vi "ideal_inverse_kinematics.vi"(11 "Pose":T1) -> (3 "Axis positions":dbl[](array[numeric]))   [LabVIEW 2011]
uses:
  <vilib>/Analysis/Matrix/Datatypes/RealMatrix.ctl
  <vilib>/Analysis/baseanly.llb/A x Vector.vi
  <vilib>/Analysis/NI_AALBase.lvlib
  <vilib>/Analysis/Matrix/NI_Matrix.lvlib
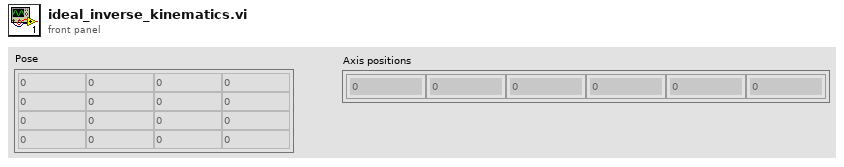
[diagram p1: front panel]
types:
  T1 = typedef "NI_Matrix.lvlib/RealMatrix.ctl" = dbl[][]
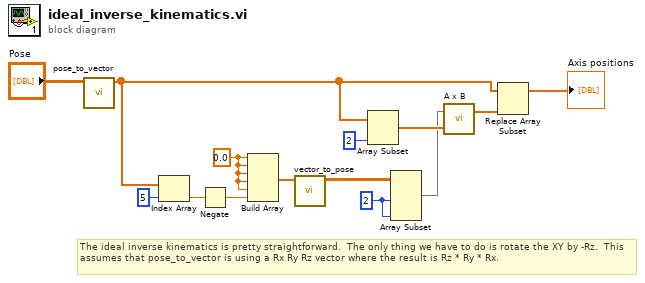
[diagram p0: block diagram]
diagram:
  w8 = 2 ("length")
  w3 = 0.0 ("element")
  # "The ideal inverse kinematics is pretty straightforward.  The only thing we have to do is rotate the XY by -Rz.  This assumes that pose_to_vector is using a Rx Ry Rz vector where the result is Rz * Ry * Rx."
  n1 = call "pose_to_vector.vi"("Pose"="Pose") -> ("Pose vector"=w13:dbl[])  [unwired: 10 in]
  n2 = Index Array(array=w13, index=5) -> (element=w5:dbl)
  n3 = Negate(x=w5) -> (-x=w6:dbl)
  n4 = Build Array(w3, w3, w3, w3, w3, w6) -> (w4:dbl[])
  n5 = call "vector_to_pose.vi"("Pose vector"=w4) -> ("Pose"=w7:T1)  [unwired: 10 in]
  n6 = Array Subset(array=w13, length=2) -> (w11:dbl[])  [unwired: 1 in]
  n7 = Array Subset(array=w7, length (row)=w8, length (col)=w8) -> (w10:T1)  [unwired: 2 in]
  n8 = call-poly <vilib>:"A x B.vi"("Vector"=w11, "A"=w10) -> ("A x Vector"=w12:dbl[])  [unwired: 1 out]
  n9 = Replace Array Subset(array=w13, new element=w12) -> (→"Axis positions":dbl[])  [unwired: 1 in]
